vi "pathfinder generate.vi"(8 "error in (no error)":errorcluster, 11 "trajectory length":i32) -> (0 "error out":errorcluster, 3 "Segments":T1[](array[typedef]))   [LabVIEW 2016, in "Pathfinder.lvlib"]
doc: "CAPI int pathfinder_generate_LabVIEW(Segment *segments);"
uses:
  Pathfinder.lvlib
  Segment.ctl
  pathfinder.dll
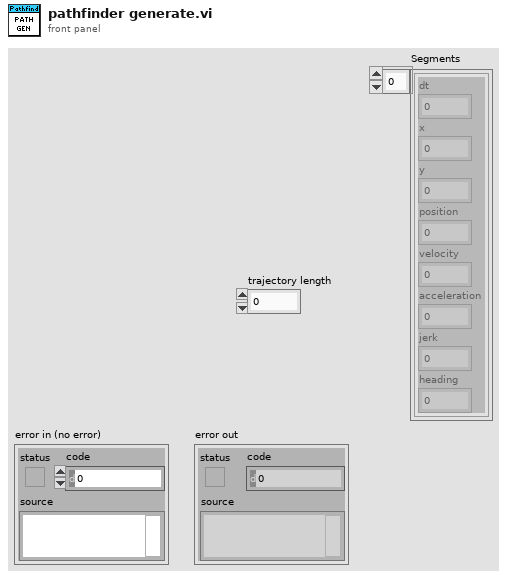
[diagram p1: front panel]
types:
  T1 = typedef "Pathfinder.lvlib/Segment.ctl" = cluster{"dt":dbl, "x":dbl, "y":dbl, "position":dbl, "velocity":dbl, "acceleration":dbl, "jerk":dbl, "heading":dbl}
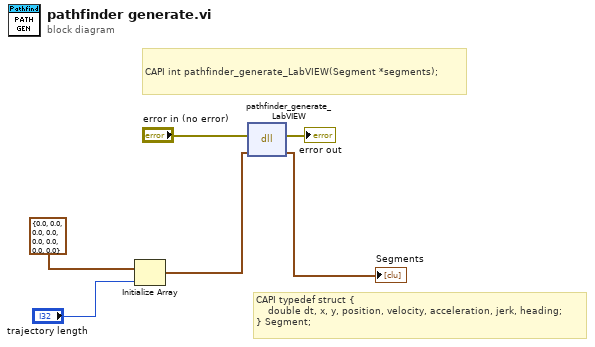
[diagram p0: block diagram]
diagram:
  # "CAPI typedef struct {\n    double dt, x, y, position, velocity, acceleration, jerk, heading;\n} Segment;"
  # "CAPI int pathfinder_generate_LabVIEW(Segment *segments);"
  n1 = Initialize Array(T1 {"dt"=0.0, "x"=0.0, "y"=0.0, "position"=0.0, "velocity"=0.0, "acceleration"=0.0, "jerk"=0.0, "heading"=0.0} ("segment"), "trajectory length") -> (w3:T1[])
  n2 = dll-call lib="C:/Users/a0272913/Documents/LabVIEW Data/Pathfinder/Pathfinder/pathfinder.*" fn="pathfinder_generate_LabVIEW"(error in="error in (no error)", "segments"=w3) -> (error out=→"error out":errorcluster, "segments"=→"Segments":T1[])  [unwired: 3 in, 1 out]
